vi "Close.vi"(8 "error in":errorcluster, 11 "Cycler in":refnum<class "Cycler.lvclass">) -> (0 "error out":errorcluster, 3 "Cycler out":refnum<class "Cycler.lvclass">)   [LabVIEW 2023, in "Cycler.lvclass"]
uses:
  Cycler.lvclass
  Cycler.lvclass/Cycler.ctl
  <vilib>/ADAS Replay HIL/AdasHilServices/AdasHilServices Fill In Error Info Ex.vi
  <vilib>/ADAS Replay HIL/AdasHilServices/AdasHilChannelServices.lvlib
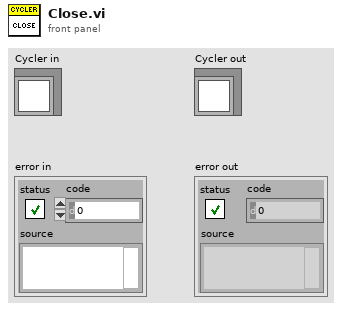
[diagram p1: front panel]
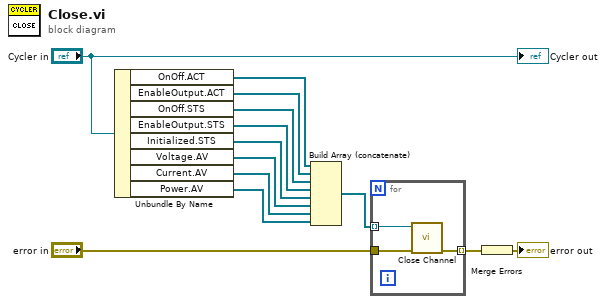
[diagram p0: block diagram]
diagram:
  n1 = Unbundle By Name("Cycler in") -> ("OnOff.ACT"=w9:refnum<k21>[], "EnableOutput.ACT"=w8:refnum<k21>[], "OnOff.STS"=w7:refnum<k21>[], "EnableOutput.STS"=w6:refnum<k21>[], "Initialized.STS"=w5:refnum<k21>[], "Voltage.AV"=w4:refnum<k21>[], "Current.AV"=w3:refnum<k21>[], "Power.AV"=w2:refnum<k21>[])
  n2 = Build Array (concatenate)(w9, w8, w7, w6, w5, w4, w3, w2) -> (w1:refnum<k21>[])
  n3 = for {
    tunnel: w1 -> [w14] mode=indexing
    tunnel: "error in" -> [w16]
    tunnel: [w15] -> w11 mode=indexing
    n4 = call <vilib>:"Close Channel.vi"("error in"=w16, "ADAS HIL Channel"=w14) -> ("error out"=w15:errorcluster)  [unwired: 9 in]
  }
  n5 = Merge Errors(w11) -> (→"error out":errorcluster)
  "Cycler out" <- "Cycler in"
